vi "RSZVB Set Port Waveguide Attenuator.vi"(6 "Attenuation (8.0)":dbl=8.0 format="%^.3e", 7 "Waveguide Attenuator (Mechanical)":i32(ring) items=["Mechanical", "Electronic"], 8 "error in (no error)":errorcluster {"code" format="%.0x"}, 9 "Port (1)":i32=1, 10 "Channel (1)":i32=1, 11 "VISA session":refnum<visa-resource-name>) -> (0 "error out":errorcluster {"code" format="%.0x"}, 3 "dup VISA session":refnum<visa-resource-name>)   [LabVIEW 2011]
doc: "This VI selects the waveguide attenuator type of the converter port <Pt> and attenuation for a converter with electronic or mechanical attenuators at port <Pt>.\n\nRemote-control command(s):\nSOURce<Ch>:POWer<Pt>:CONVerter:TRANsfer:ATTenuator MECHanical |\nELECtronic\nSOURce<Ch>:POWer<Pt>:CONVerter:TRANsfer:ELECtronic:MATTenuation\n<attenuation>\nSOURce<Ch>:POWer<Pt>:CONVerter:TRANsfer:MECHanical:ATTenuation\n<attenuation>"
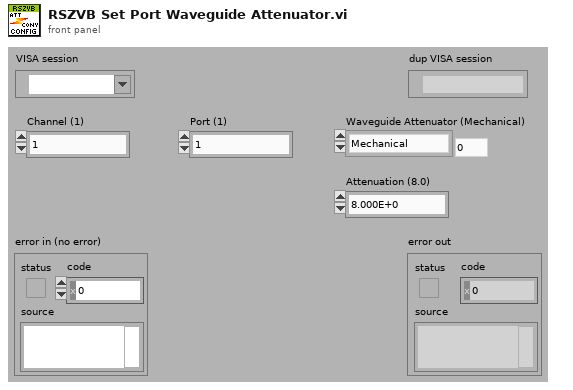
[diagram p1: front panel]
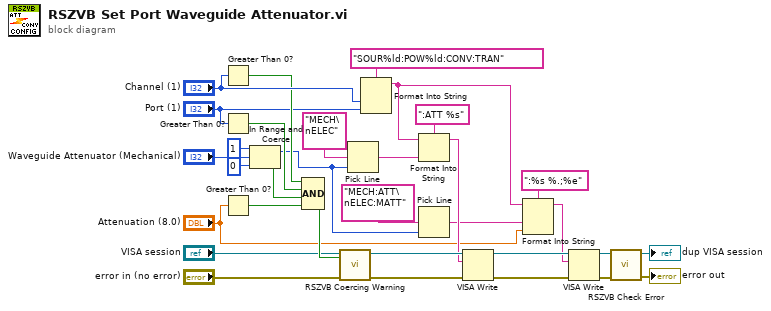
[diagram p0: block diagram]
diagram:
  n1 = Greater Than 0?(x="Channel (1)") -> (x > 0?=w21:bool)
  n2 = Greater Than 0?(x="Port (1)") -> (x > 0?=w18:bool)
  n3 = Greater Than 0?(x="Attenuation (8.0)") -> (x > 0?=w2:bool)
  n4 = In Range and Coerce(upper limit=1, x="Waveguide Attenuator (Mechanical)", lower limit=0) -> (coerced(x)=w11:i32, In Range?=w28:bool)
  n5 = Compound Arithmetic op=AND(w21, w18, w28, w2) -> (w27:bool)
  n6 = call "RSZVB Coercing Warning.vi"("In Range?"=w27, "error in (no error)"="error in (no error)", "VISA session"="VISA session") -> ("error out"=w29:errorcluster, "dup VISA session"=w30:refnum<visa-resource-name>)  [unwired: 7 in]
  n7 = Pick Line(multi-line string="MECH\nELEC", line index=w11) -> (output string=w16:string)  [unwired: 1 in]
  n8 = Format Into String(format string="SOUR%ld:POW%ld:CONV:TRAN", "Channel (1)", "Port (1)") -> (resulting string=w13:string)  [unwired: 2 in, 1 out]
  n9 = Format Into String(format string=":ATT %s", initial string=w13, w16) -> (resulting string=w15:string)  [unwired: 1 in, 1 out]
  n10 = Pick Line(multi-line string="MECH:ATT\nELEC:MATT", line index=w11) -> (output string=w10:string)  [unwired: 1 in]
  n11 = VISA Write(VISA resource name=w30, write buffer=w15, error in (no error)=w29) -> (VISA resource name out=w8:refnum<visa-resource-name>, error out=w9:errorcluster)  [unwired: 1 out]
  n12 = Format Into String(format string=":%s %.;%e", initial string=w13, w10, "Attenuation (8.0)") -> (resulting string=w7:string)  [unwired: 1 in, 1 out]
  n13 = VISA Write(VISA resource name=w8, write buffer=w7, error in (no error)=w9) -> (VISA resource name out=w6:refnum<visa-resource-name>, error out=w5:errorcluster)  [unwired: 1 out]
  n14 = call "RSZVB Check Error.vi"("error in (no error)"=w5, "VISA session"=w6) -> ("error out"=→"error out":errorcluster, "dup VISA session"=→"dup VISA session":refnum<visa-resource-name>)  [unwired: 8 in]
